vi "Change Filter.vi"(8 "error in":errorcluster, 10 "crdFilt":bool, 11 "CRDS in":refnum<class "CRDS.lvclass">) -> (0 "error out":errorcluster, 3 "CRDS out":refnum<class "CRDS.lvclass">)   [LabVIEW 2011, in "CRDS.lvclass"]
uses:
  CRDS.lvclass
  CRDS.lvclass/CRDS.ctl
  Reusable/Switch/Switch.lvclass
  <vilib>/DAQmx/write.llb/DAQmx Write (Digital 1D Bool NChan 1Samp 1Line).vi
  <vilib>/DAQmx/miscellaneous.llb/DAQmx Fill In Error Info.vi
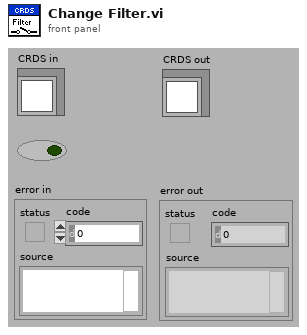
[diagram p1: front panel]
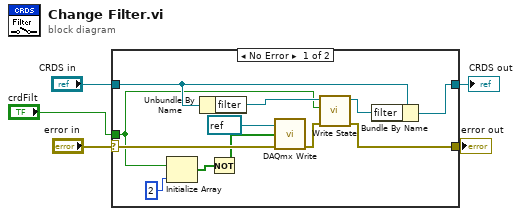
[diagram p0: block diagram]
diagram:
  n1 = case shown="No Error" "error in" {
    selector: "error in" -> [w17 w19]
    tunnel: [w11 w19] -> w4
    tunnel: [w13 w18] -> w2
    tunnel: "CRDS in" -> [w15 w18]
    tunnel: "crdFilt" -> [w9 _]
    frame No Error {
      n2 = Initialize Array(w9, 2 ("dimension size")) -> (w8:bool[])
      n3 = Unbundle By Name(w15) -> ("filter"=w16:refnum<class "Switch.lvclass">)
      n4 = Not(x=w8) -> (.not. x?=w7:bool[])
      n5 = call-poly <vilib>:"DAQmx Write.vi"("task/channels in"=refnum<k21> refnum, "data"=w7, "error in"=w17) -> ("error out"=w12:errorcluster)  [unwired: 10 in, 2 out]
      n6 = call-dynamic "Write State.vi"("error in (no error)"=w12, "State"=w9, "Switch in"=w16) -> ("error out"=w11:errorcluster, "Switch out"=w14:refnum<class "Switch.lvclass">)  [unwired: 7 in]
      n7 = Bundle By Name(cluster=w15, "filter"=w14) -> (w13:refnum<class "CRDS.lvclass">)
    }
    frame Error {
    }
  }
  "error out" <- w4
  "CRDS out" <- w2
